vi "Evaluate Default Trigger (Array).vi"(8 "error in (no error)":errorcluster, 10 "Trigger Data":dbl[](array[numeric]), 11 "Default Trigger in":refnum<class "Default Trigger.lvclass">) -> (0 "error out":errorcluster, 1 "Trigger indices":i32[](array[numeric]), 2 "Trigger":bool, 3 "Default Trigger out":refnum<class "Default Trigger.lvclass">)   [LabVIEW 2015, in "Default Trigger.lvclass"]
doc: "Evaluates the trigger data and returns whether the specified trigger condition was met."
uses:
  Default Trigger.lvclass
  Default Trigger.lvclass/Default Trigger.ctl
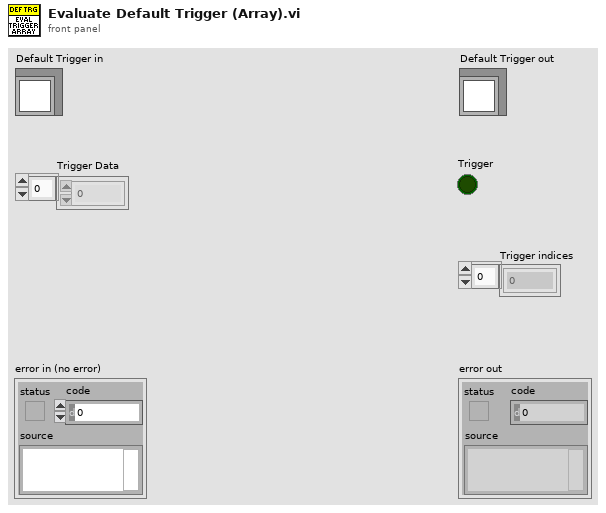
[diagram p1: front panel]
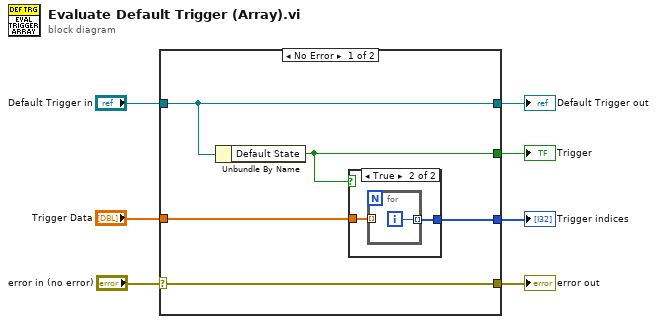
[diagram p0: block diagram]
diagram:
  n1 = case shown="No Error" "error in (no error)" {
    selector: "error in (no error)" -> [w11 w16]
    tunnel: "Default Trigger in" -> [w12 w17]
    tunnel: [w10 _] -> w6
    tunnel: [w12 w17] -> w4
    tunnel: [w11 w16] -> w3
    tunnel: "Trigger Data" -> [w9 _]
    tunnel: [w8 _] -> w1
    frame No Error {
      n2 = Unbundle By Name(w12) -> ("Default State"=w10:bool)
      n3 = case shown="True" w10 {
        tunnel: w9 -> [_ w14]
        tunnel: [_ w13] -> w8
        frame False {
        }
        frame True {
          n4 = for {
            tunnel: w14 -> [_] mode=indexing
            tunnel: [w15] -> w13 mode=indexing
            i -> [w15]
          }
        }
      }
    }
    frame Error {
    }
  }
  "error out" <- w3
  "Default Trigger out" <- w4
  "Trigger" <- w6
  "Trigger indices" <- w1
